vi "Filter (G3)-Create QBPN.vi"(0 "Filter":T1={"Type"=enum."Lowpass", "CF (kHz)"=0.0, "BW (kHz)"=0.0, "Cascade"=FALSE, "Quadrature"=FALSE, "Scale Factor"=0.0, "Stages"=[], "Class"=enum."Elliptic", "Order"=0, "BWUnits"=enum."Linear"} {"Stages"."IIR Filter"."Forward Coefficients" format="%.4f"; "Stages"."IIR Filter"."Reverse Coefficients" format="%.4f"}, 7 "Npts":i32=128, 11 "Omega (t)":dbl[](array[numeric])) -> (4 "Filter (out)":T1={"Type"=enum."Lowpass", "CF (kHz)"=0.0, "BW (kHz)"=0.0, "Cascade"=FALSE, "Quadrature"=FALSE, "Scale Factor"=0.0, "Stages"=[], "Class"=enum."Elliptic", "Order"=0, "BWUnits"=enum."Linear"} {"Stages"."IIR Filter"."Forward Coefficients" format="%.4f"; "Stages"."IIR Filter"."Reverse Coefficients" format="%.4f"}, 8 "BP noise":dbl[](array[numeric]))   [LabVIEW 2020]
doc: "Create a token of bandpass noise using the quadrature filter method."
uses:
  XControls/Filter (G3)/Filter Data.ctl
  XControls/Filter (G3)/Filter Type.ctl
  Filter VIs/Filter-Bandwidth Units.ctl
  <vilib>/Analysis/3filter.llb/IIR Cascade Filter with I.C. (DBL).vi
  <vilib>/Analysis/NI_AALBase.lvlib
  XControls/Filter (G3)/Filter (G3).xctl
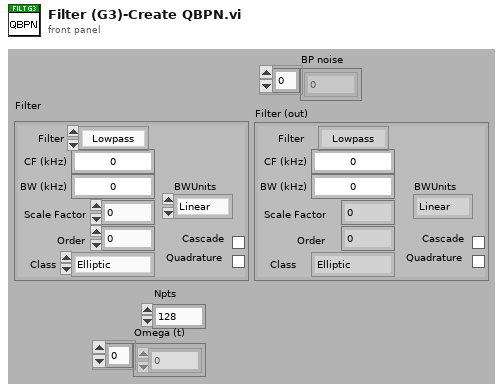
[diagram p1: front panel]
types:
  T1 = typedef "Filter (G3).xctl/Filter Data.ctl" = cluster{"Type":T2, "CF (kHz)":dbl, "BW (kHz)":dbl, "Cascade":bool, "Quadrature":bool, "Scale Factor":dbl, "Stages":cluster{"IIR Filter":cluster{"filter structure":enum32{"IIR 2nd Order", "IIR 4th Order"}, "Reverse Coefficients":dbl[], "Forward Coefficients":dbl[]}, "State":dbl[]}[], "Class":enum16{"Elliptic", "Butterworth"}, "Order":i32, "BWUnits":T3}
  T2 = typedef "Filter (G3).xctl/Filter Type.ctl" = enum16{"OFF", "Lowpass", "Highpass", "Bandpass", "Bandstop"}
  T3 = typedef "Filter-Bandwidth Units.ctl" = enum16{"Linear", "Octaves", "Min-Max"}
  T4 = cluster{"IIR Filter":cluster{"filter structure":enum32{"IIR 2nd Order", "IIR 4th Order"}, "Reverse Coefficients":dbl[], "Forward Coefficients":dbl[]}, "State":dbl[]}[]
  T5 = cluster{"IIR Filter":cluster{"filter structure":enum32{"IIR 2nd Order", "IIR 4th Order"}, "Reverse Coefficients":dbl[], "Forward Coefficients":dbl[]}, "State":dbl[]}
  T6 = cluster{"filter structure":enum32{"IIR 2nd Order", "IIR 4th Order"}, "Reverse Coefficients":dbl[], "Forward Coefficients":dbl[]}
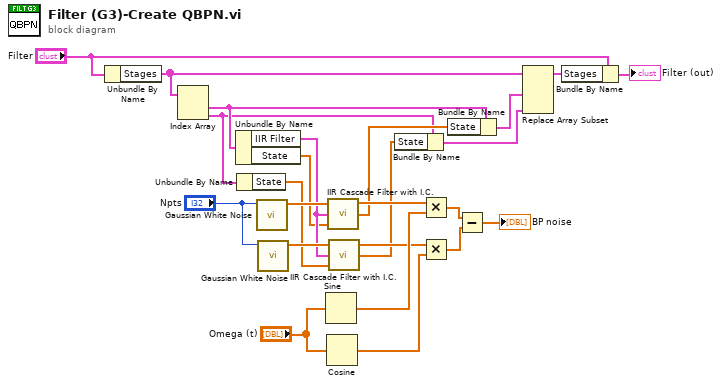
[diagram p0: block diagram]
diagram:
  n1 = Unbundle By Name("Filter") -> ("Stages"=w6:T4)
  n2 = Index Array(array=w6) -> (element #1=w10:T5, element #2=w8:T5)  [unwired: 2 in]
  n3 = Unbundle By Name(w10) -> ("IIR Filter"=w13:T6, "State"=w12:dbl[])
  n4 = Unbundle By Name(w8) -> ("State"=w11:dbl[])
  n5 = call <vilib>:"Gaussian White Noise.vi"("samples"="Npts") -> ("Gaussian noise pattern"=w23:dbl[])  [unwired: 9 in, 1 out]
  n6 = call <vilib>:"Gaussian White Noise.vi"("samples"="Npts") -> ("Gaussian noise pattern"=w24:dbl[])  [unwired: 9 in, 1 out]
  n7 = Sine(x="Omega (t)") -> (sin(x)=w22:dbl[])
  n8 = Cosine(x="Omega (t)") -> (cos(x)=w20:dbl[])
  n9 = call-poly <vilib>:"IIR Cascade Filter with I.C..vi"("Initial Filter State"=w12, "IIR Filter Cluster"=w13, "X"=w23) -> ("Final Filter State"=w9:dbl[], "Filtered X"=w17:dbl[])  [unwired: 1 out]
  n10 = call-poly <vilib>:"IIR Cascade Filter with I.C..vi"("Initial Filter State"=w11, "IIR Filter Cluster"=w13, "X"=w24) -> ("Final Filter State"=w7:dbl[], "Filtered X"=w21:dbl[])  [unwired: 1 out]
  n11 = Bundle By Name(cluster=w8, "State"=w7) -> (w4:T5)
  n12 = Multiply(x=w17, y=w22) -> (x*y=w19:dbl[])
  n13 = Multiply(x=w21, y=w20) -> (x*y=w18:dbl[])
  n14 = Bundle By Name(cluster=w10, "State"=w9) -> (w5:T5)
  n15 = Subtract(x=w19, y=w18) -> (x-y=→"BP noise":dbl[])
  n16 = Replace Array Subset(array=w6, new element #1=w5, new element #2=w4) -> (w2:T4)  [unwired: 2 in]
  n17 = Bundle By Name(cluster="Filter", "Stages"=w2) -> (→"Filter (out)":T1)
